vi "create.request.vi"(7 "Time Stamp (now: system time)":timestamp format="%<%x %.3X>T", 8 "error in":errorcluster, 9 "Type":enum16{"INFO", "FLAG", "ERROR", "SUCCESS"}(ring), 10 "Name":string, 11 "assets":refnum<class "asset.lvclass">[](array[class])) -> (0 "error out":errorcluster, 3 "request":string)   [LabVIEW 2020, in "event.lvclass"]
uses:
  asset/asset.lvclass
  asset/asset.lvclass/asset.ctl
  88b4df77-45d7-451c-ac61-e829d33da7cc.vi
  f3b2abde-4779-4471-9147-3371a6e54b37.vi
  asset/rid.get.vi
  352cc468-aba9-4bd5-96da-7e448382693f.vi
  <vilib>/LabVIEW Open Source Project/Epoch Date & Time/epoch.UNIX/Epoch.UNIX.lvclass
  C:/Program Files/National Instruments/LabVIEW 2020/vi.lib/LabVIEW Open Source Project/Epoch Date & Time/epoch/Epoch.lvclass
  <vilib>/LabVIEW Open Source Project/Epoch Date & Time/Get Epoch Time.vi
  <vilib>/JDP Science/JSONtext/Variant to JSON Text.vi
  <vilib>/JDP Science/JSONtext/LVClass Serializer/JSONtext LVClass Serializer.lvclass
  event.lvclass
  event.lvclass/event.ctl
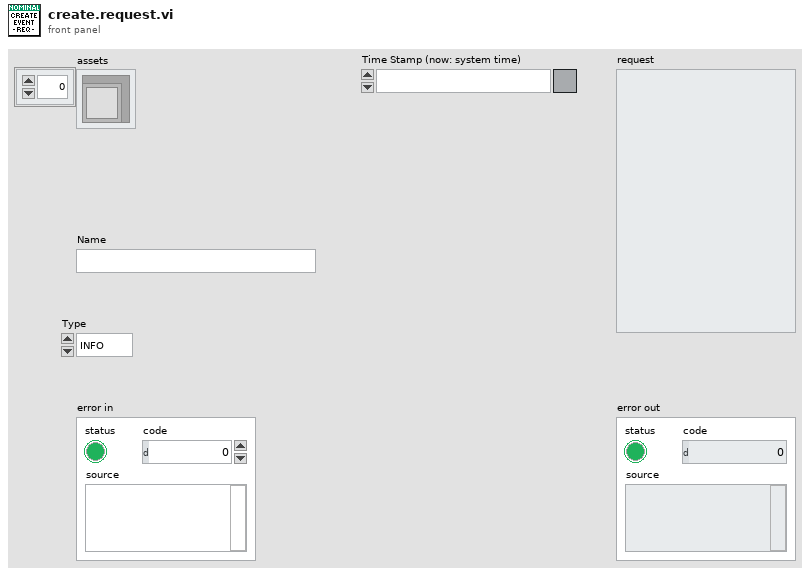
[diagram p1: front panel]
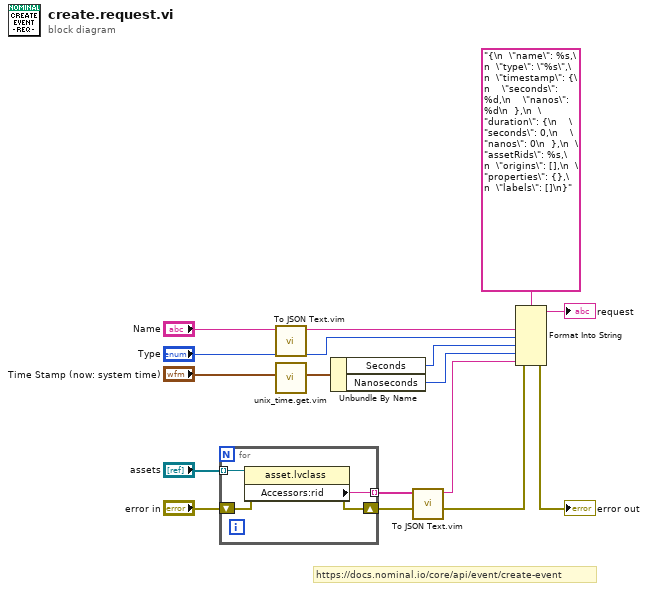
[diagram p0: block diagram]
diagram:
  # "https://docs.nominal.io/core/api/event/create-event"
  n1 = for {
    tunnel: "assets" -> [w20] mode=indexing
    tunnel: [w19] -> w9 mode=indexing
    shift-right: [w18] -> w4
    shift-left: "error in" -> [w17]
    n2 = property class="asset.lvclass"(reference=w20, error in=w17) -> (error out=w18:errorcluster, "Accessors:rid"=w19:string)  [unwired: 1 out]
  }
  n3 = call "To JSON Text.vim"("Anything"="Name") -> ("<JSON>"=w1:string)  [unwired: 9 in, 1 out]
  n4 = call "unix_time.get.vim"("Time Stamp (empty: now) [single or array]"="Time Stamp (now: system time)") -> ("UNIX Timestamp"=w13:cluster{"Seconds":i64, "Nanoseconds":i64})  [unwired: 10 in]
  n5 = Unbundle By Name(w13) -> ("Seconds"=w12:i64, "Nanoseconds"=w11:i64)
  n6 = call "To JSON Text.vim"("error in (no error)"=w4, "Anything"=w9) -> ("error out"=w7:errorcluster, "<JSON>"=w8:string)  [unwired: 8 in]
  n7 = Format Into String(format string="{\n  \"name\": %s,\n  \"type\": \"%s\",\n  \"timestamp\": {\n    \"seconds\": %d,\n    \"nanos\": %d\n  },\n  \"duration\": {\n    \"seconds\": 0,\n    \"nanos\": 0\n  },\n  \"assetRids\": %s,\n  \"origins\": [],\n  \"properties\": {},\n  \"labels\": []\n}", error in=w7, w1, "Type", w12, w11, w8) -> (resulting string=→"request":string, error out=→"error out":errorcluster)  [unwired: 1 in]
